vi "Command Picture.vi"(5 "Unused":bool, 7 "Feedback State":T1, 10 "Command State":T1, 11 "Command Pictures":T3) -> (2 "Command Picture":T2)   [LabVIEW 2020, in "VolatusGUI.lvlib" / "2WayValve.lvclass"]
uses:
  2WayValve.lvclass
  Channel State.ctl
  Command Pictures.ctl
  Picture.ctl
  2WayValve.lvclass/2WayValve.ctl
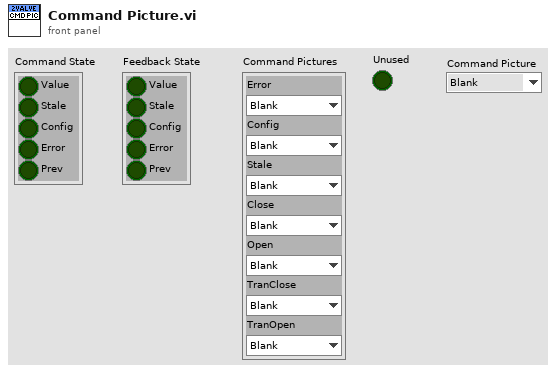
[diagram p1: front panel]
types:
  T1 = typedef "VolatusGUI.lvlib/2WayValve.lvclass/Channel State.ctl" = cluster{"Value":bool, "Stale":bool, "Config":bool, "Error":bool, "Prev":bool}
  T2 = typedef "VolatusGUI.lvlib/2WayValve.lvclass/Picture.ctl" = enum16{"Blank", "OutClose", "OutOpen", "OutTranClose", "OutTranOpen", "OutConfig", "OutStale", "OutError", "InClose", "InOpen", "InTranClose", "InTranOpen", "InConfig", "InStale", "InError", "EnOff", "EnOn", "EnConfig", "EnStale", "EnError"}
  T3 = typedef "VolatusGUI.lvlib/2WayValve.lvclass/Command Pictures.ctl" = cluster{"Error":T2, "Config":T2, "Stale":T2, "Close":T2, "Open":T2, "TranClose":T2, "TranOpen":T2}
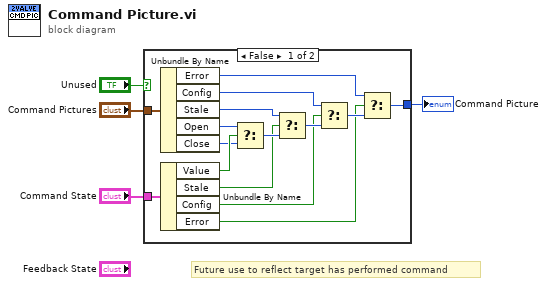
[diagram p0: block diagram]
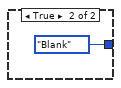
[diagram p2: hidden frame]
diagram:
  # "Future use to reflect target has performed command"
  n1 = case shown="False" "Unused" {
    tunnel: "Command State" -> [w19 _]
    tunnel: "Command Pictures" -> [w18 _]
    tunnel: [w5 Picture."Blank" ("Close")] -> w2
    frame False {
      n2 = Unbundle By Name(w18) -> ("Error"=w7:T2, "Config"=w8:T2, "Stale"=w13:T2, "Open"=w15:T2, "Close"=w16:T2)
      n3 = Unbundle By Name(w19) -> ("Value"=w17:bool, "Stale"=w12:bool, "Config"=w10:bool, "Error"=w6:bool)
      n4 = Select(t=w15, s=w17, f=w16) -> (s? t:f=w14:T2)
      n5 = Select(t=w13, s=w12, f=w14) -> (s? t:f=w11:T2)
      n6 = Select(t=w8, s=w10, f=w11) -> (s? t:f=w9:T2)
      n7 = Select(t=w7, s=w6, f=w9) -> (s? t:f=w5:T2)
    }
    frame True {
    }
  }
  "Command Picture" <- w2
